vi "FactoryCreate.vi"(8 "Error In":errorcluster, 10 "InstrumentConfig":T1, 11 "reference in":refnum<class "VdInstrument.lvclass">) -> (0 "Error Out":errorcluster, 3 "reference out":refnum<class "VdInstrument.lvclass">)   [LabVIEW 2020, in "VdInstrument.lvclass"]
uses:
  VdInstrument.lvclass
  InstrumentConfig.ctl
  InstrumentType.ctl
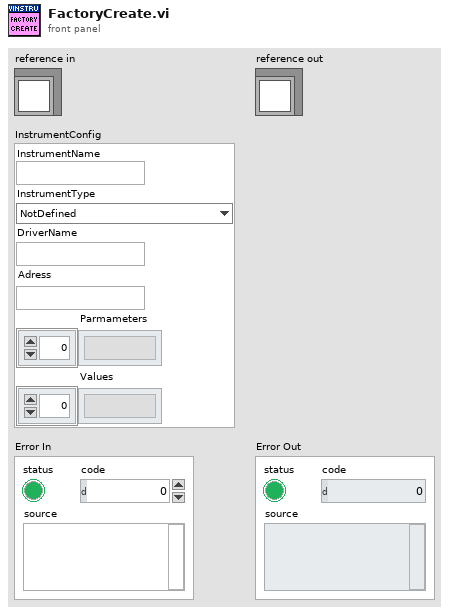
[diagram p1: front panel]
types:
  T1 = typedef "VdInstrument.lvclass/InstrumentConfig.ctl" = cluster{"InstrumentName":string, "InstrumentType":T2, "DriverName":string, "Adress":string, "Parmameters":string[], "Values":string[]}
  T2 = typedef "VdInstrument.lvclass/InstrumentType.ctl" = enum16{"NotDefined", "AirflowController", "AnalogInput", "AnalogOutput", "AutoCollimator", "BeamProfiler", "DMM", "DigitalControl", "DigitalInput", "DisplacementSensor", "Encoder", "ForceSensor", "FrequencyCounter", "FunctionGenerator", "GelDispensingRobot", "GlueDispenser", "Hexapod", "IRCamera", "ImageGenerator", "LabelPrinter", "LightController", "LightIndicator", "Load", "Multimeter", "OpticalAttenuatorPowerMeter", "OpticalChannelMonitor", "OpticalLaser", "OpticalPolarizationController", "OpticalPowerAttenuator", "OpticalPowerMeter", "OpticalSpectrumAnalyzer", "PDLMeter", "PolarisationScrambler", "PolarizationAnalyzer", "PositionSensitiveDetector", "PowerSupply", "PressureController", "Robot", "SLRCamera", "ScrewdriverController", "SignalAnalyzer", "SignalGenerator", "SixAxisStage", "SolderingStation", "SpectrumAnalyzer", "StepperMotor", "Stirrer", "SweptWavelengthSystem", "Switch", "TemperatureChamber", "TemperatureController", "TemperatureSensor", "TunableLaser", "UVCuring", "UsbHub", "VisionCamera", "WavelengthMeter", "WeldingLaser"}
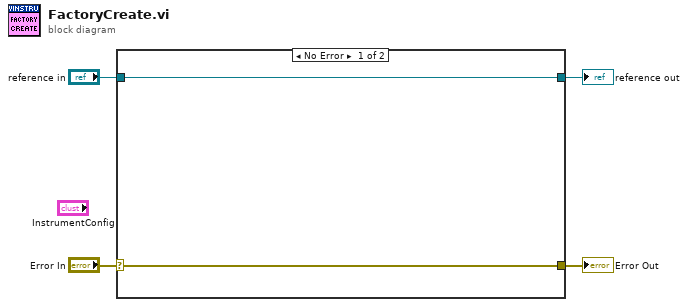
[diagram p0: block diagram]
diagram:
  n1 = case shown="No Error" "Error In" {
    selector: "Error In" -> [w5 w8]
    tunnel: [w5 w8] -> w3
    tunnel: [w6 w7] -> w1
    tunnel: "reference in" -> [w6 w7]
    frame No Error {
    }
    frame Error {
    }
  }
  "Error Out" <- w3
  "reference out" <- w1
